vi "Temp Folder--constant.vi"() -> (3 "Temp Folder":path)   [LabVIEW 2025]
doc: "This constant defines the temporary folder for the project execution."
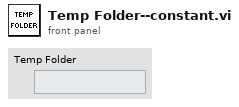
[diagram p1: front panel]
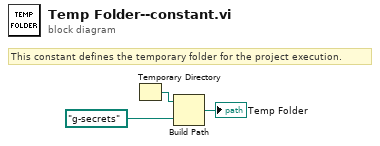
[diagram p0: block diagram]
diagram:
  # "This constant defines the temporary folder for the project execution."
  n1 = Temporary Directory() -> (w3:path)
  n2 = Build Path(base path=w3, name or relative path=path "g-secrets" ("Test Folder")) -> (appended path=→"Temp Folder":path)
